vi "Request_str_str.vi"(0 "reference in":T1, 5 "method":string, 7 "params":refnum<class "JSON Null.lvclass">, 9 "id":string, 11 "error in (no error)":errorcluster) -> (4 "reference out":T1, 6 "reponse":string, 15 "error out":errorcluster)   [LabVIEW 2017, in "JSON_RPC_client.lvlib"]
uses:
  JSON_RPC_client.lvlib
  reference.ctl
  <vilib>/httpClient/ClientHandle.ctl
  <vilib>/NI/JSON Support for LabVIEW/JSON Data Classes/JSON Datatype/JSON Null.lvclass
  <vilib>/NI/JSON Support for LabVIEW/JSON Data Classes/JSON Object/New JSON Object (Empty).vi
  <vilib>/NI/JSON Support for LabVIEW/JSON Data Classes/JSON Object/Insert Key Value Pair.vi
  <vilib>/NI/JSON Support for LabVIEW/JSON Data Classes/JSON Object/Insert Key Value Pair (Single String).vi
  <vilib>/NI/JSON Support for LabVIEW/JSON Data Classes/JSON Object/Insert Key Value Pair (Single).vi
  <vilib>/httpClient/POSTBuffer.vi
  <vilib>/NI/JSON Support for LabVIEW/JSON Data Classes/JSON Object/Set Object Parameters XNode/Set Object Parameters.xnode
  <vilib>/NI/JSON Support for LabVIEW/JSON Data Classes/JSON Object/JSON Object.lvclass
  <vilib>/httpClient/LabVIEWHTTPClient.lvlib
  <vilib>/NI/JSON Support for LabVIEW/JSON Data Classes/JSON Helper/JSON Helper.lvclass
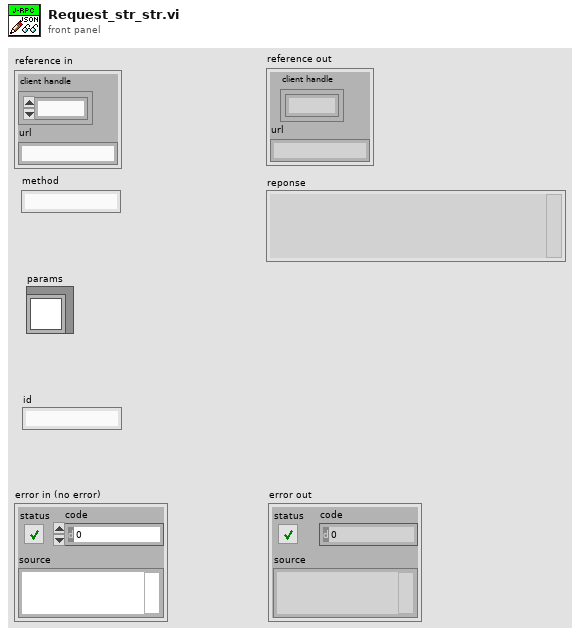
[diagram p1: front panel]
types:
  T1 = typedef "JSON_RPC_client.lvlib/reference.ctl" = cluster{"client handle":T2, "url":string}
  T2 = typedef "LabVIEWHTTPClient.lvlib/ClientHandle.ctl" = refnum<k1>
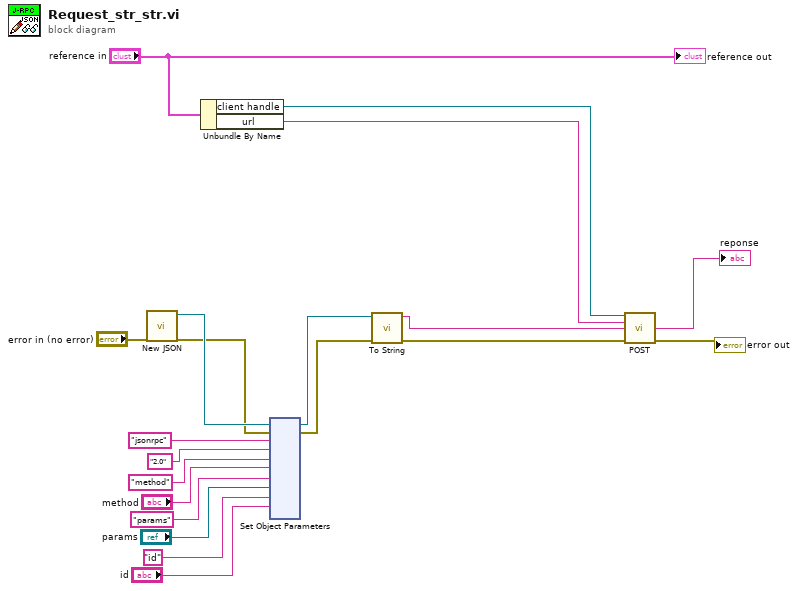
[diagram p0: block diagram]
diagram:
  n1 = call-poly <vilib>:"New JSON.vi"("error in (no error)"="error in (no error)") -> ("error out"=w5:errorcluster, "JSON Object out"=w14:refnum<class "JSON Object.lvclass">)  [unwired: 9 in]
  n2 = Unbundle By Name("reference in") -> ("client handle"=w17:T2, "url"=w16:string)
  n3 = xnode "Set Object Parameters"("key"="jsonrpc" ("Name"), "key"="method" ("Name"), "key"="params" ("Name"), "key"="id" ("Name"), "parameter"="2.0" ("String"), "parameter"="method", "parameter"="params", "parameter"="id", "JSON Object In"=w14, "error in"=w5) -> ("JSON Object Out"=w4:refnum<class "JSON Object.lvclass">, "error out"=w3:errorcluster)  [unwired: 4 out]
  n4 = call-dynamic "To String.vi"("error in (no error)"=w3, "JSON Object in"=w4) -> ("error out"=w1:errorcluster, "String"=w2:string)  [unwired: 8 in]
  n5 = call-poly <vilib>:"POST.vi"("client handle"=w17, "url"=w16, "buffer"=w2, "error in (no error)"=w1) -> ("body"=→"reponse":string, "error out"=→"error out":errorcluster)  [unwired: 8 in, 2 out]
  "reference out" <- "reference in"
